vi "Is Armed.vi"(8 "error in (no error)":errorcluster, 11 "RP Instrument in":refnum<class "RP Instrument.lvclass">) -> (0 "error out":errorcluster, 1 "Finished":bool, 2 "Armed":bool, 3 "RP Instrument out":refnum<class "RP Instrument.lvclass">, 4 "Status response":u32=1 format="0x%x (%d)")   [LabVIEW 2020, in "RP Instrument.lvclass"]
uses:
  RP Instrument.lvclass
  RP Status Offsets.ctl
  RP Instrument.lvclass/RP Instrument.ctl
  RP Config Offsets.ctl
  RP Communicator/RP Communicator.lvclass
panel:
  out "Writer address max":u32=1 format="0x%x (%d)"
  out "Record start max":u32=1 format="0x%x (%d)"
  out "Actual record length":u32=1 format="0x%x (%d)"
  out "Record length":u32=1 format="0x%x (%d)"
  out "Writer address":u32=1 format="0x%x (%d)"
  out "Record start":u32=1 format="0x%x (%d)"
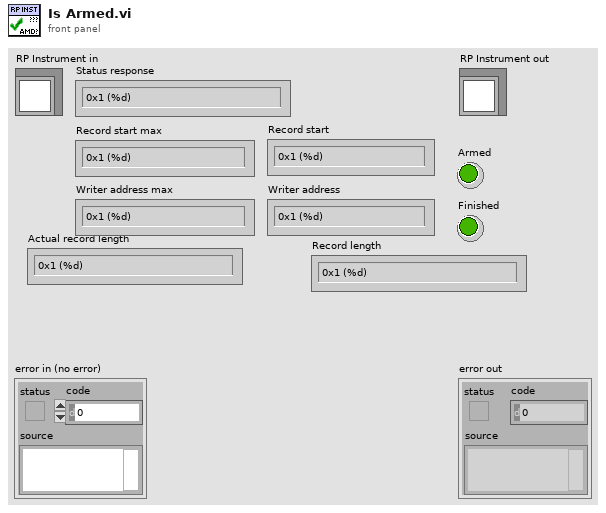
[diagram p1: front panel]
types:
  T1 = typedef "RP Status Offsets.ctl" = u16
  T2 = typedef "RP Config Offsets.ctl" = u16
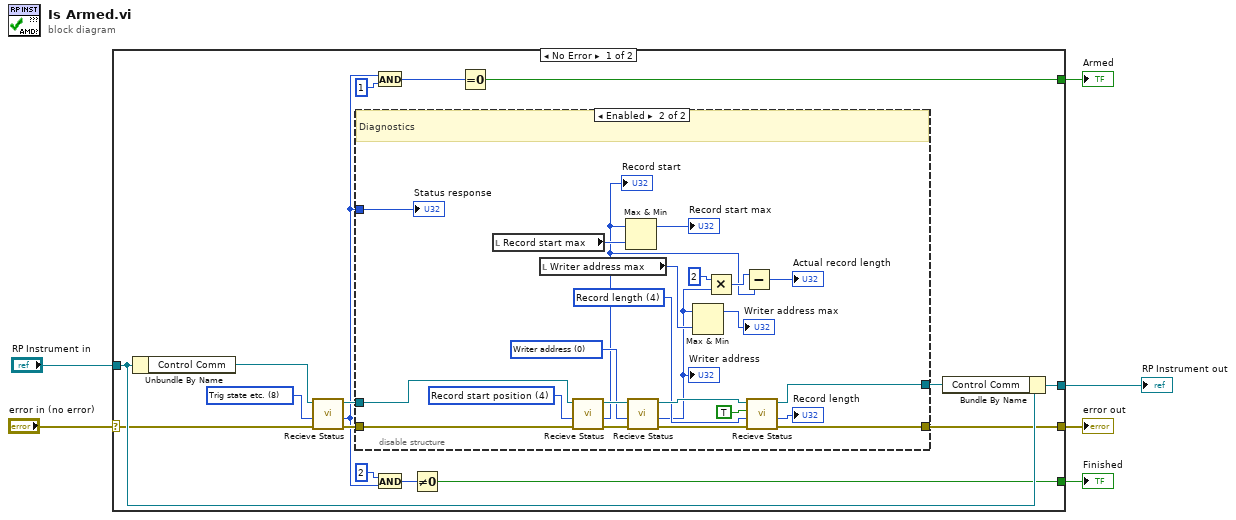
[diagram p0: block diagram]
diagram:
  n1 = case shown="No Error" "error in (no error)" {
    selector: "error in (no error)" -> [w18 w49]
    tunnel: [w8 w49] -> w5
    tunnel: [w19 w48] -> w3
    tunnel: "RP Instrument in" -> [w22 w48]
    tunnel: [w13 _] -> w2
    tunnel: [w12 _] -> w1
    frame No Error {
      w17 = T1 8 items=["Writer address"=0, "Record start position"=4, "Trig state etc."=8, "RxFIFO counter"=24, "TxFIFO counter"=28] ("Status offsets")
      n2 = Unbundle By Name(w22) -> ("Control Comm"=w21:refnum<class "RP Communicator.lvclass">)
      n3 = call-dynamic "Recieve Status.vi"("error in (no error)"=w18, "Status offset"=w17, "RP Communicator in"=w21) -> ("error out"=w9:errorcluster, "Status response"=w7:u32, "RP Communicator out"=w11:refnum<class "RP Communicator.lvclass">)  [unwired: 6 in]
      n4 = disable-structure shown="Enabled" {
        disable-tunnel: w11 -> [w24 w46]
        disable-tunnel: w9 -> [w23 w47]
        disable-tunnel: [w24 w38] -> w10
        disable-tunnel: [w23 w40] -> w8
        disable-tunnel: w7 -> [_ w32]
        frame Disabled {
        }
        frame Enabled {
          w36 = T2 4 items=["Config flags"=0, "Record length"=4, "Frequency"=8, "Decimation"=12, "LED"=16, "DDS delay"=28] ("Config offsets")
          w41 = T1 0 items=["Writer address"=0, "Record start position"=4, "Trig state etc."=8, "RxFIFO counter"=24, "TxFIFO counter"=28] ("Status offsets")
          w45 = T1 4 items=["Writer address"=0, "Record start position"=4, "Trig state etc."=8, "RxFIFO counter"=24, "TxFIFO counter"=28] ("Status offsets")
          # "Diagnostics"
          n5 = local read "Record start max"() -> (w31:u32)
          n6 = local read "Writer address max"() -> (w29:u32)
          n7 = call-dynamic "Recieve Status.vi"("error in (no error)"=w47, "Status offset"=w45, "RP Communicator in"=w46) -> ("error out"=w42:errorcluster, "Status response"=w25:u32, "RP Communicator out"=w44:refnum<class "RP Communicator.lvclass">)  [unwired: 6 in]
          "Record start" <- w25
          n8 = Max & Min(x=w25, y=w31) -> (max(x,y)=→"Record start max":u32)  [unwired: 1 out]
          n9 = call-dynamic "Recieve Status.vi"("error in (no error)"=w42, "Status offset"=w41, "RP Communicator in"=w44) -> ("error out"=w43:errorcluster, "Status response"=w27:u32, "RP Communicator out"=w39:refnum<class "RP Communicator.lvclass">)  [unwired: 6 in]
          "Writer address" <- w27
          n10 = Max & Min(x=w27, y=w29) -> (max(x,y)=→"Writer address max":u32)  [unwired: 1 out]
          n11 = Multiply(x=u32 2, y=w27) -> (x*y=w26:u32)
          n12 = Subtract(x=w26, y=w25) -> (x-y=→"Actual record length":u32)
          n13 = call-dynamic "Recieve Status.vi"("error in (no error)"=w43, "Status offset"=w36, "Read config instead"=TRUE, "RP Communicator in"=w39) -> ("error out"=w40:errorcluster, "Status response"=→"Record length":u32, "RP Communicator out"=w38:refnum<class "RP Communicator.lvclass">)  [unwired: 5 in]
          "Status response" <- w32
        }
      }
      n14 = And(x=w7, y=u32 1) -> (x .and. y?=w20:u32)
      n15 = And(x=u32 2 ("y"), y=w7) -> (x .and. y?=w14:u32)
      n16 = Not Equal To 0?(x=w14) -> (x != 0?=w13:bool)
      n17 = Equal To 0?(x=w20) -> (x = 0?=w12:bool)
      n18 = Bundle By Name(cluster=w22, "Control Comm"=w10) -> (w19:refnum<class "RP Instrument.lvclass">)
    }
    frame Error {
    }
  }
  "error out" <- w5
  "RP Instrument out" <- w3
  "Finished" <- w2
  "Armed" <- w1
